vi "Async.Engine.Reconfigure.vi"(8 "error in":errorcluster, 10 "Compiled.InlineAsync.Settings":T3 {"Read"."Refs"."Data Reference" format="%.0x"; "Write"."Refs"."Data Reference" format="%.0x"; "ReadWrite"."Refs" format="%.0x"}, 11 "Async in":refnum<class "VS Inline Async API.lvclass">) -> (0 "error out":errorcluster, 2 "Data Access Engine":refnum<class "Data Access Engine.lvclass">, 3 "Async out":refnum<class "VS Inline Async API.lvclass">)   [LabVIEW 2023, in "VS Inline Async API.lvlib" / "VS Inline Async API.lvclass"]
uses:
  VS Inline Async API.lvclass
  <vilib>/NI VeriStand/Custom Device API/Block Data Reference.ctl
  <vilib>/NI VeriStand/Custom Device API/Data Reference.ctl
  _Data Access Engine/Data Access Engine/Data Access Engine.lvclass
  VS Inline Async API.lvclass/VS Inline Async API.ctl
  <vilib>/NI VeriStand/Custom Device API/Custom Device API.lvlib
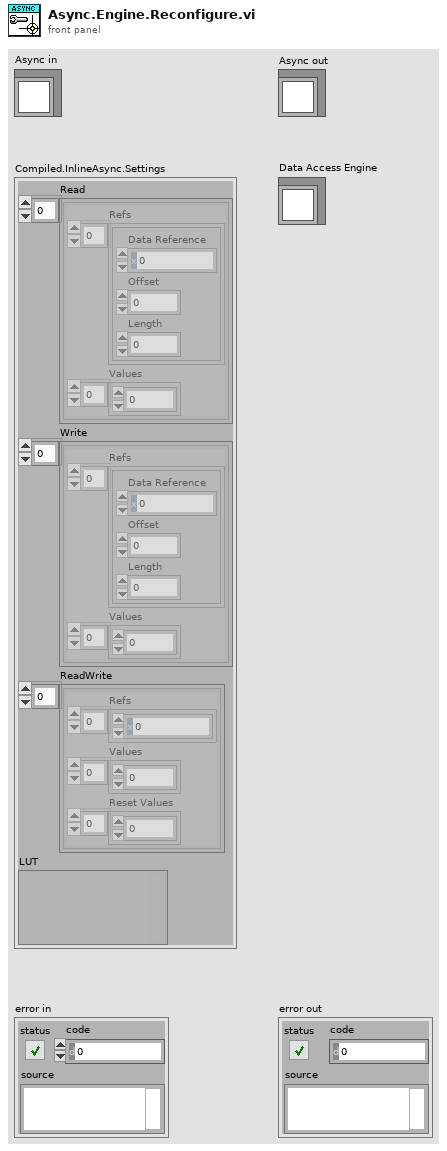
[diagram p1: front panel]
types:
  T1 = typedef "Custom Device API.lvlib/Block Data Reference.ctl" = cluster{"Data Reference":T2, "Offset":u64, "Length":u64}
  T2 = typedef "Custom Device API.lvlib/Data Reference.ctl" = i32
  T3 = cluster{"Read":cluster{"Refs":T1[], "Values":dbl[]}[], "Write":cluster{"Refs":T1[], "Values":dbl[]}[], "ReadWrite":cluster{"Refs":T2[], "Values":dbl[], "Reset Values":dbl[]}[], "LUT":variant}
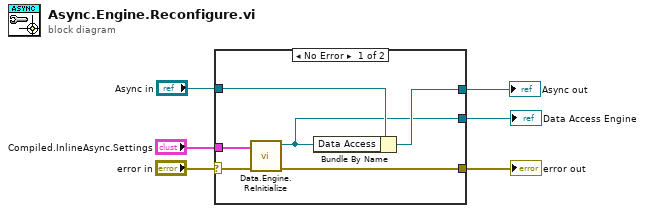
[diagram p0: block diagram]
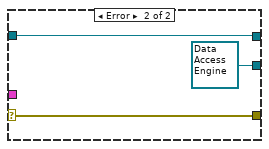
[diagram p2: hidden frame]
diagram:
  n1 = case shown="No Error" "error in" {
    selector: "error in" -> [w11 w15]
    tunnel: "Compiled.InlineAsync.Settings" -> [w10 _]
    tunnel: "Async in" -> [w9 w14]
    tunnel: [w8 w14] -> w2
    tunnel: [w7 refnum<class "Data Access Engine.lvclass"> refnum ("Data Access Engine")] -> w1
    tunnel: [w12 w15] -> w6
    frame No Error {
      n2 = call "Data.Engine.ReInitialize.vi"("error in"=w11, "Compiled.InlineAsync.Settings"=w10) -> ("error out"=w12:errorcluster, "Data Access Engine"=w7:refnum<class "Data Access Engine.lvclass">)  [unwired: 8 in]
      n3 = Bundle By Name(cluster=w9, "Data Access"=w7) -> (w8:refnum<class "VS Inline Async API.lvclass">)
    }
    frame Error {
    }
  }
  "Async out" <- w2
  "Data Access Engine" <- w1
  "error out" <- w6
